vi "Open Connection_SALDATA.vi"(8 "error in (no error)":errorcluster, 9 "Control 2":T1, 10 "topicName":string) -> (0 "error out":errorcluster, 3 "topicRef":cluster{"topicName":string, "type":refnum<vi>})   [LabVIEW 2012]
uses:
  SALTypedefs/Control 2.ctl
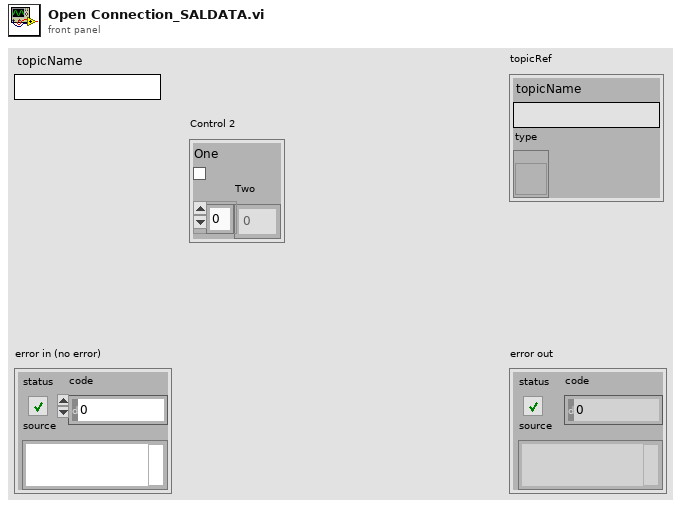
[diagram p1: front panel]
types:
  T1 = typedef "Control 2.ctl" = cluster{"One":bool, "Two":i32[]}
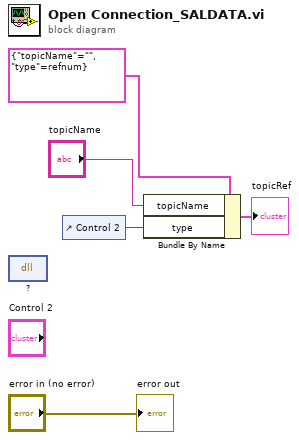
[diagram p0: block diagram]
diagram:
  n1 = dll-call lib="?" fn="?"() -> ()  [unwired: 4 in, 2 out]
  n2 = control-ref of="Control 2"() -> (w2:refnum<vi>)
  n3 = Bundle By Name(cluster=cluster{"topicName":string, "type":refnum<vi>} {"topicName"="", "type"=refnum} ("topicRef"), "topicName"="topicName", "type"=w2) -> (→"topicRef":cluster{"topicName":string, "type":refnum<vi>})
  "error out" <- "error in (no error)"
